vi "Read VISA Refnum.vi"(8 "error in (no error)":errorcluster, 11 "Driver in":refnum<class "Driver.lvclass">) -> (0 "error out":errorcluster, 2 "VISA Refnum":refnum<visa-resource-name>, 3 "Driver out":refnum<class "Driver.lvclass">)   [LabVIEW 2023, in "Driver.lvlib" / "Driver.lvclass"]
uses:
  Driver.lvclass
  Driver.lvclass/Driver.ctl
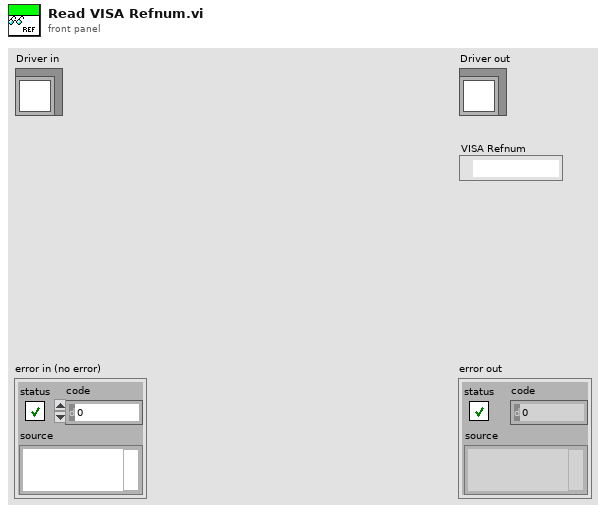
[diagram p1: front panel]
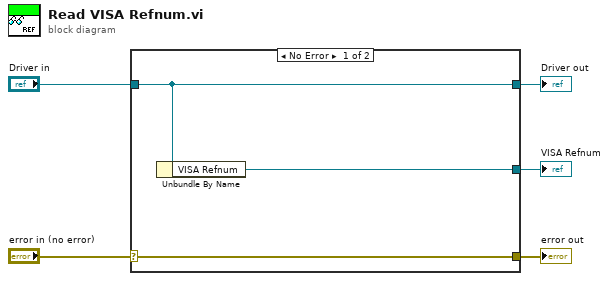
[diagram p0: block diagram]
diagram:
  n1 = case shown="No Error" "error in (no error)" {
    selector: "error in (no error)" -> [w8 w9]
    tunnel: [w8 w9] -> w4
    tunnel: [w7 w10] -> w2
    tunnel: "Driver in" -> [w7 w10]
    tunnel: [w6 _] -> w1
    frame No Error {
      n2 = Unbundle By Name(w7) -> ("VISA Refnum"=w6:refnum<visa-resource-name>)
    }
    frame Error {
    }
  }
  "error out" <- w4
  "Driver out" <- w2
  "VISA Refnum" <- w1
